vi "Test In-Place Array Row Replace.vi"() -> ()   [LabVIEW 2015]
panel:
  out "Probe Data Array in 3":u8[][](array[numeric])
  in  "Probe Data Array in 2":u8[](array[numeric])=[100, 101, 102, 103, 104]
  in  "Probe Data Array in":u8[][](array[numeric])=[[0, 1, 2, 3, 4], [10, 11, 12, 13, 14], [20, 21, 22, 23, 24], [30, 31, 32, 33, 34], [40, 41, 42, 43, 44]]
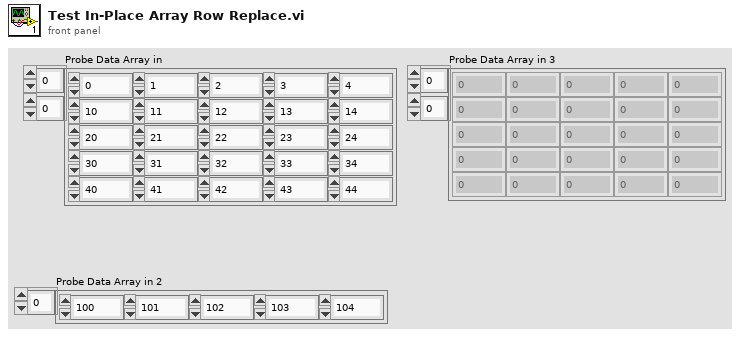
[diagram p1: front panel]
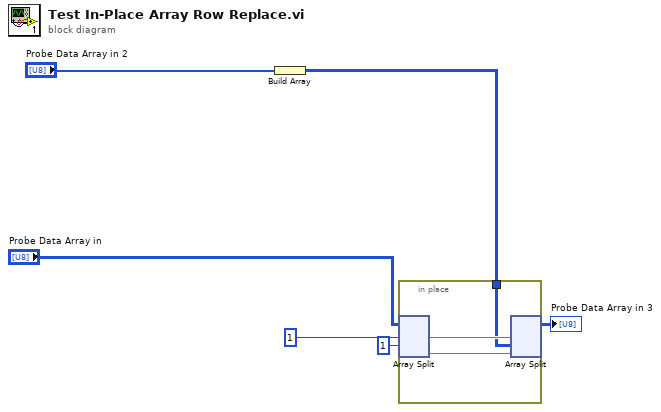
[diagram p0: block diagram]
diagram:
  n1 = Build Array("Probe Data Array in 2") -> (w4:u8[][])
  n2 = in-place {
    in-place-border: w4 -> [w7]
    n3 = in-place-split #1("Probe Data Array in", 1, 1) -> (w9:u8[][], w8:u8[][])  [unwired: 1 out]
    n4 = in-place-split #1(w9, w7, w8) -> (→"Probe Data Array in 3":u8[][])  [unwired: 2 out]
  }
